vi "Result Data Update the Self.vi"(8 "error in (no error)":errorcluster, 10 "Report Data":T1={"Schema"="", "Test Socket"="", "Start Test Cycle"="", "Stop Test Cycle"="", "Test Mode"="", "Frame Type"="fe_frame_log"}, 11 "Signal Analysis in":refnum<class "Signal Analysis.lvclass">) -> (0 "error out":errorcluster, 3 "Signal Analysis out":refnum<class "Signal Analysis.lvclass">)   [LabVIEW 2023, in "Data Analysis.lvlib" / "Signal Analysis.lvlib" / "Signal Analysis.lvclass"]
uses:
  Signal Analysis.lvclass
  Control/Report.ctl
  Signal Analysis.lvclass/Signal Analysis.ctl
  Data Analysis.lvlib
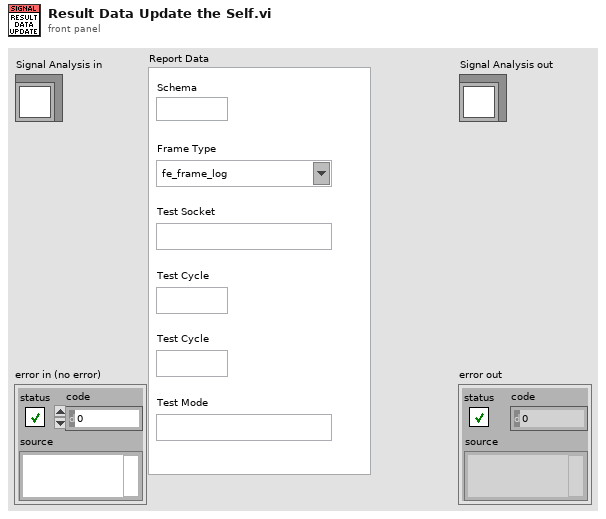
[diagram p1: front panel]
types:
  T1 = typedef "Data Analysis.lvlib/Report.ctl" = cluster{"Schema":string, "Test Socket":string, "Start Test Cycle":string, "Stop Test Cycle":string, "Test Mode":string, "Frame Type":string}
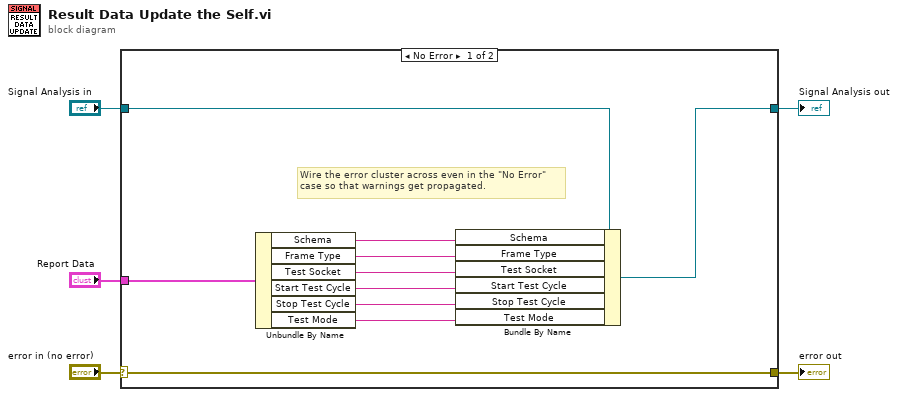
[diagram p0: block diagram]
diagram:
  n1 = case shown="No Error" "error in (no error)" {
    selector: "error in (no error)" -> [w15 w17]
    tunnel: [w15 w17] -> w4
    tunnel: [w9 w16] -> w2
    tunnel: "Signal Analysis in" -> [w7 w16]
    tunnel: "Report Data" -> [w8 _]
    frame No Error {
      # "Wire the error cluster across even in the \"No Error\"\ncase so that warnings get propagated."
      n2 = Unbundle By Name(w8) -> ("Schema"=w6:string, "Frame Type"=w14:string, "Test Socket"=w13:string, "Start Test Cycle"=w12:string, "Stop Test Cycle"=w11:string, "Test Mode"=w10:string)
      n3 = Bundle By Name(cluster=w7, "Schema"=w6, "Frame Type"=w14, "Test Socket"=w13, "Start Test Cycle"=w12, "Stop Test Cycle"=w11, "Test Mode"=w10) -> (w9:refnum<class "Signal Analysis.lvclass">)
    }
    frame Error {
    }
  }
  "error out" <- w4
  "Signal Analysis out" <- w2
